vi "DIAG_STM Set Meta Data.vi"   [LabVIEW 2015, in "Diagnostics Addon Engine.lvlib"]
doc: "Assigns the meta data cluster associated with this STM session."
uses:
  Diagnostics Addon Engine.lvlib
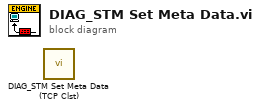
[diagram p0: block diagram]
diagram:
  n1 = call "DIAG_STM Set Meta Data (TCP Clst).vi"() -> ()  [unwired: 10 in, 2 out]
